vi "Calculate_(101)-(11)_Global_Cost_F()-1.vi"(5 "[IN] Still connect\ned tracks in group":T1, 6 "[IN] Max angle":dbl, 7 "[IN] Subtracks":T2(array[cluster]), 8 "error IN":errorcluster, 9 "[IN] Areas particles\nPrimary Detected":dbl[][](array[numeric]), 10 "[IN] Primary \n(X,Y) Detected":dbl[][](array[numeric]), 11 "[IN] Cost function":i8[](array[numeric])) -> (0 "error OUT":errorcluster, 3 "[OUT] Cost function":i8[](array[numeric]))   [LabVIEW 2013]
uses:
  <vilib>/Analysis/NI_AALBase.lvlib
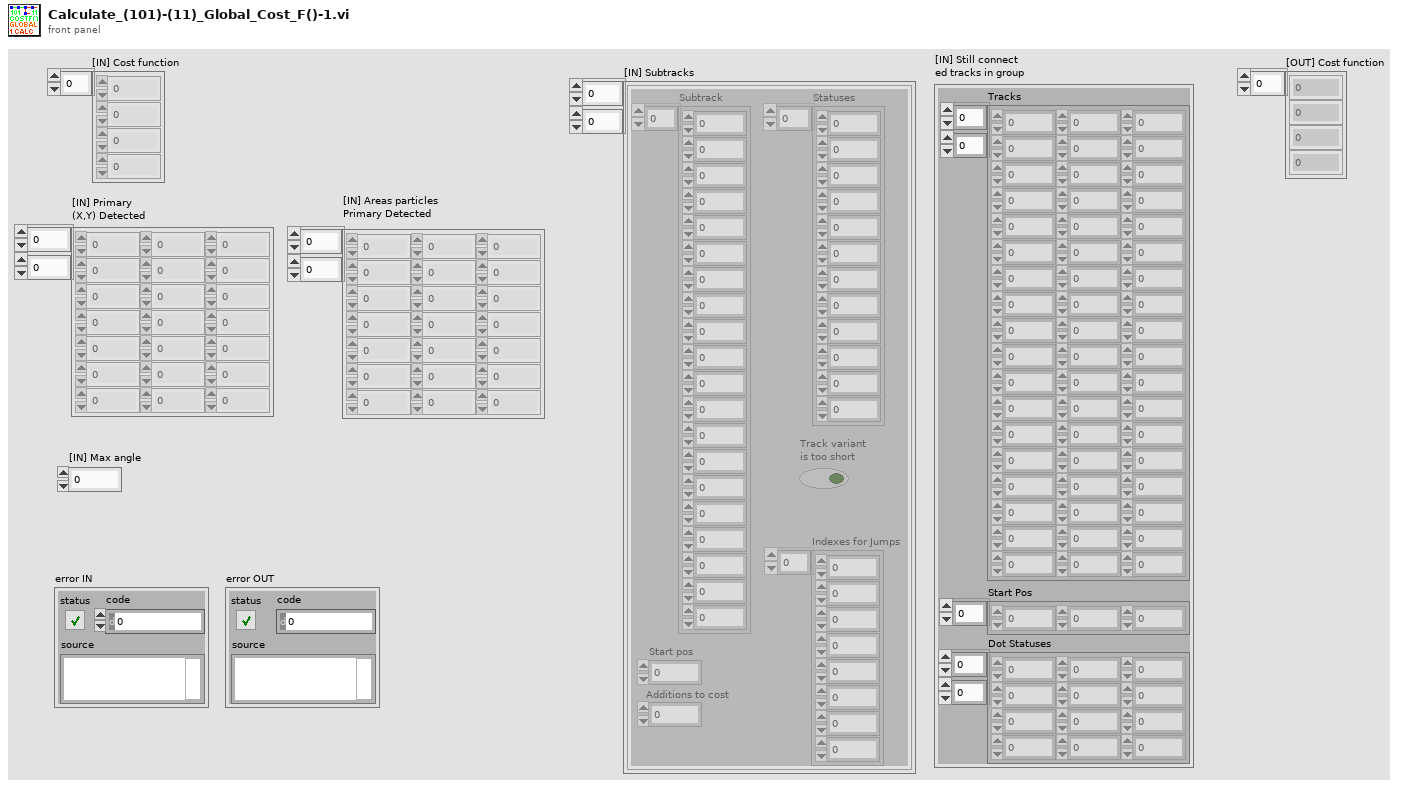
[diagram p1: front panel]
types:
  T1 = cluster{"Tracks":dbl[][], "Start Pos":i32[], "Dot Statuses":i16[][]}
  T2 = cluster{"Subtrack":dbl[], "Statuses":i16[], "Start pos":i32, "Additions to cost":i32, "Track variant \nis too short":bool, "Indexes for Jumps":i32[]}[][]
  T3 = cluster{"Subtrack":dbl[], "Statuses":i16[], "Start pos":i32, "Additions to cost":i32, "Track variant \nis too short":bool, "Indexes for Jumps":i32[]}[]
  T4 = cluster{"Subtrack":dbl[], "Statuses":i16[], "Start pos":i32, "Additions to cost":i32, "Track variant \nis too short":bool, "Indexes for Jumps":i32[]}
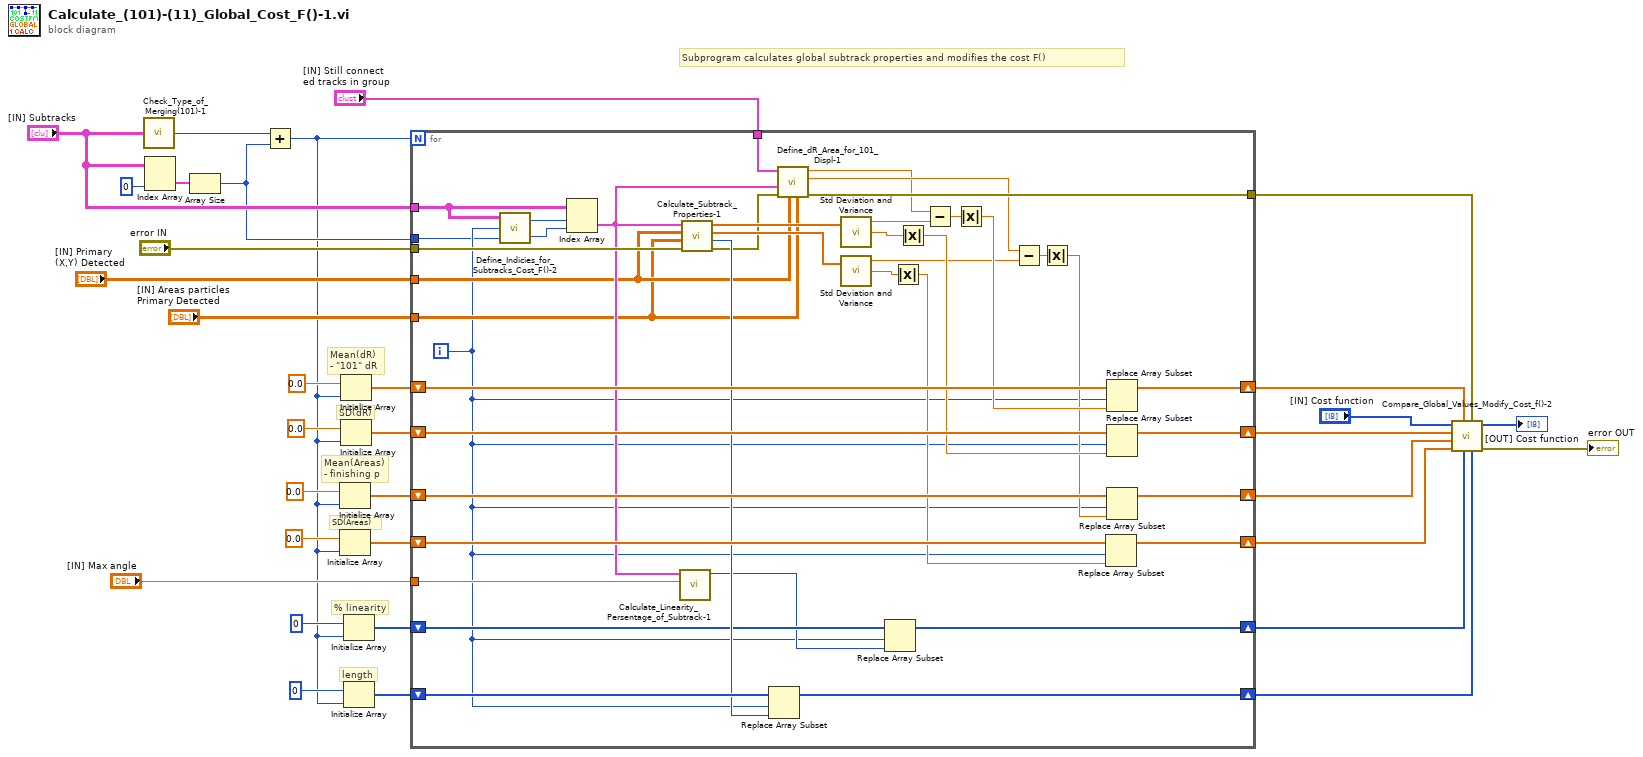
[diagram p0: block diagram]
diagram:
  # "Subprogram calculates global subtrack properties and modifies the cost F()"
  # "Mean(Areas)\n- finishing p"
  # "SD(Areas)"
  # "% linearity"
  # "length"
  # "Mean(dR)\n- \"101\" dR"
  # "SD(dR)"
  n1 = call "Check_Type_of_Merging(101)-1.vi"("[IN] Subtracks"="[IN] Subtracks") -> ("[OUT] # of Additional Costs"=w2:i32)
  n2 = Index Array(array="[IN] Subtracks", index (col)=0 ("disabled index (col)")) -> (element=w32:T3)  [unwired: 1 in]
  n3 = Array Size(array=w32) -> (size(s)=w3:i32)
  n4 = Add(x=w2, y=w3) -> (x+y=w1:i32)
  n5 = Initialize Array(0.0, w1) -> (w20:dbl[])
  n6 = Initialize Array(0.0, w1) -> (w19:dbl[])
  n7 = Initialize Array(0.0, w1) -> (w29:dbl[])
  n8 = Initialize Array(0.0, w1) -> (w28:dbl[])
  n9 = Initialize Array(u8 0, w1) -> (w15:u8[])
  n10 = Initialize Array(u8 0, w1) -> (w18:u8[])
  n11 = for {
    N: w1 -> [_]
    tunnel: "[IN] Subtracks" -> [w38]
    shift-right: [w69] -> w13
    shift-left: w29 -> [w72]
    shift-right: [w68] -> w11
    shift-left: w28 -> [w71]
    tunnel: "error IN" -> [w74]
    tunnel: "[IN] Primary \n(X,Y) Detected" -> [w42]
    tunnel: "[IN] Areas particles\nPrimary Detected" -> [w41]
    shift-right: [w62] -> w10
    shift-left: w20 -> [w67]
    shift-right: [w65] -> w9
    shift-left: w19 -> [w66]
    shift-right: [w57] -> w5
    shift-left: w18 -> [w59]
    tunnel: "[IN] Still connect\ned tracks in group" -> [w46]
    tunnel: "[IN] Max angle" -> [w50]
    shift-right: [w47] -> w6
    shift-left: w15 -> [w49]
    tunnel: [w43] -> w14
    tunnel: w3 -> [w36]
    i -> [w37]
    n12 = call "Define_Indicies_for_Subtracks_Cost_F()-2.vi"("[IN] Number of Rows"=w36, "[IN] Current index"=w37, "[IN] Subtracks"=w38) -> ("[OUT] Column \n# for Subtrack"=w34:i32, "[OUT] Row # \nfor Subtrack"=w35:i32)
    n13 = Index Array(array=w38, index (row)=w35, index (col)=w34) -> (element=w45:T4)
    n14 = call "Calculate_Linearity_Persentage_of_Subtrack-1.vi"("[IN] Max angle"=w50, "[IN] Subtrack"=w45) -> ("[OUT] Track Linearity in %"=w48:u8)  [unwired: 5 in]
    n15 = call "Calculate_Subtrack_Properties-1.vi"("error IN"=w74, "[IN] Areas particles\nPrimary Detected"=w41, "[IN] Primary \n(X,Y) Detected"=w42, "[IN] Subtrack"=w45) -> ("error OUT"=w44:errorcluster, "[OUT] Length of track"=w58:u8, "[OUT] Areas"=w70:dbl[], "[OUT] dR (displ)"=w73:dbl[])  [unwired: 2 in]
    n16 = Replace Array Subset(array=w59, new element=w58, index=w37) -> (w57:u8[])
    n17 = call "Define_dR_Area_for_101_Displ-1.vi"("[IN] Areas particles\nPrimary Detected"=w41, "[IN] Primary \n(X,Y) Detected"=w42, "error IN"=w44, "[IN] Subtrack"=w45, "[IN] Still connect\ned tracks in group"=w46) -> ("error OUT"=w43:errorcluster, "[OUT] Area of  \"101\" \ndestination point"=w40:dbl, "[OUT] dR for 101 \ndisplacement"=w39:dbl)  [unwired: 4 in]
    n18 = call <vilib>:"Std Deviation and Variance.vi"("X"=w73) -> ("mean"=w56:dbl, "standard deviation"=w64:dbl)  [unwired: 1 in, 1 out]
    n19 = call <vilib>:"Std Deviation and Variance.vi"("X"=w70) -> ("mean"=w53:dbl, "standard deviation"=w61:dbl)  [unwired: 1 in, 1 out]
    n20 = Replace Array Subset(array=w49, new element=w48, index=w37) -> (w47:u8[])
    n21 = Absolute Value(x=w61) -> (abs(x)=w60:dbl)
    n22 = Absolute Value(x=w64) -> (abs(x)=w63:dbl)
    n23 = Subtract(x=w39, y=w56) -> (x-y=w55:dbl)
    n24 = Absolute Value(x=w55) -> (abs(x)=w54:dbl)
    n25 = Subtract(x=w40, y=w53) -> (x-y=w52:dbl)
    n26 = Absolute Value(x=w52) -> (abs(x)=w51:dbl)
    n27 = Replace Array Subset(array=w66, new element=w60, index=w37) -> (w65:dbl[])
    n28 = Replace Array Subset(array=w72, new element=w54, index=w37) -> (w69:dbl[])
    n29 = Replace Array Subset(array=w71, new element=w63, index=w37) -> (w68:dbl[])
    n30 = Replace Array Subset(array=w67, new element=w51, index=w37) -> (w62:dbl[])
  }
  n31 = call "Compare_Global_Values_Modify_Cost_f()-2.vi"("[IN] Lengths"=w5, "error IN"=w14, "[IN] Linearity"=w6, "[IN] Array of Mean\n(dR) - Problem dR"=w13, "[IN] SD(Areas)"=w9, "[IN] Array of Mean(Areas)\n - Problem finish Area"=w10, "[IN] SD(dR)"=w11, "[IN] Cost function"="[IN] Cost function") -> ("error OUT"=→"error OUT":errorcluster, "[OUT] Cost function"=→"[OUT] Cost function":i8[])  [unwired: 2 in]
